vi "pmove.vi"(7 "rel move in abs mode":bool, 8 "error in (no error)":errorcluster, 9 "mode (0: rel; 1: abs)":enum16{"relative", "absolute"}(ring), 10 "distance in display unit":dbl, 11 "Motor in":refnum<class "Motor.lvclass">) -> (0 "error out":errorcluster, 3 "Motor out":refnum<class "Motor.lvclass">)   [LabVIEW 2016, in "Hardware.lvlib" / "Motor.lvlib" / "Motor.lvclass"]
uses:
  <userlib>/Common Components/Hardware/Motor/Motor/Motor.lvclass
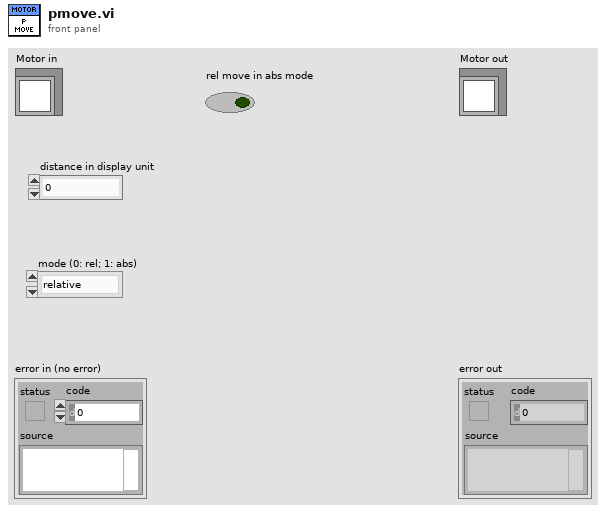
[diagram p1: front panel]
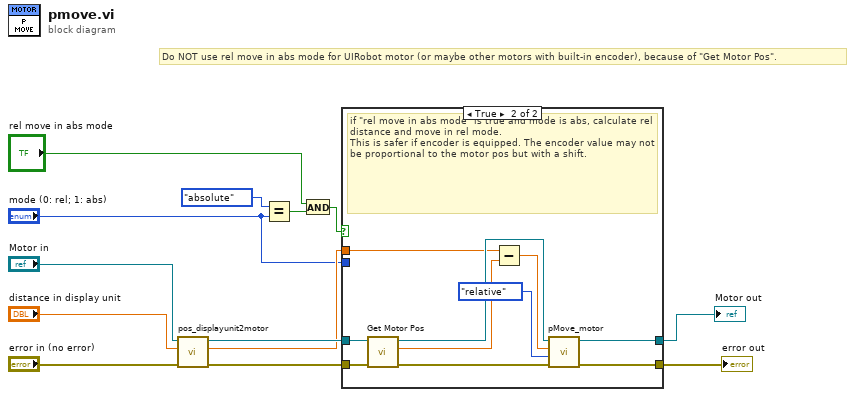
[diagram p0: block diagram]
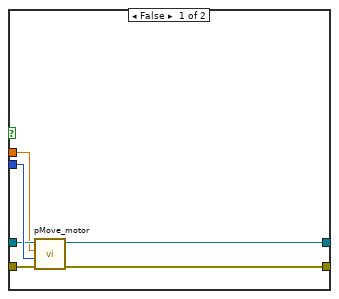
[diagram p2: hidden frame]
diagram:
  # "Do NOT use rel move in abs mode for UIRobot motor (or maybe other motors with built-in encoder), because of \"Get Motor Pos\"."
  n1 = call <userlib>:"pos_displayunit2motor.vi"("error in (no error)"="error in (no error)", "pos in display unit"="distance in display unit", "Motor in"="Motor in") -> ("error out"=w8:errorcluster, "pos in motor (pulses)"=w6:dbl, "Motor out"=w7:refnum<class "Motor.lvclass">)  [unwired: 6 in]
  n2 = Equal?(x=enum16{"relative", "absolute"}."absolute" ("y"), y="mode (0: rel; 1: abs)") -> (x = y?=w4:bool)
  n3 = And(x="rel move in abs mode", y=w4) -> (x .and. y?=w5:bool)
  n4 = case shown="True" w5 {
    tunnel: [w19 w28] -> w12
    tunnel: [w18 w25] -> w11
    tunnel: "mode (0: rel; 1: abs)" -> [w17 _]
    tunnel: w8 -> [w16 w24]
    tunnel: w7 -> [w15 w27]
    tunnel: w6 -> [w14 w23]
    frame False {
      n5 = call-dynamic "pMove_motor.vi"("error in (no error)"=w16, "mode (0: rel; 1: abs)"=w17, "distance (pulses)"=w14, "CCD in"=w15) -> ("error out"=w19:errorcluster, "CCD out"=w18:refnum<class "Motor.lvclass">)  [unwired: 6 in]
    }
    frame True {
      # "if \"rel move in abs mode\" is true and mode is abs, calculate rel distance and move in rel mode.\nThis is safer if encoder is equipped. The encoder value may not be proportional to the motor pos but with a shift."
      n6 = call-dynamic "Get Motor Pos.vi"("error in (no error)"=w24, "Motor in"=w27) -> ("error out"=w29:errorcluster, "motor pos (pulse)"=w22:dbl, "Motor out"=w26:refnum<class "Motor.lvclass">)  [unwired: 7 in]
      n7 = Subtract(x=w23, y=w22) -> (x-y=w21:dbl)
      n8 = call-dynamic "pMove_motor.vi"("error in (no error)"=w29, "mode (0: rel; 1: abs)"=enum16{"relative", "absolute"}."relative", "distance (pulses)"=w21, "CCD in"=w26) -> ("error out"=w28:errorcluster, "CCD out"=w25:refnum<class "Motor.lvclass">)  [unwired: 6 in]
    }
  }
  "error out" <- w12
  "Motor out" <- w11
